vi "Path.vi"() -> (7 "path":T1)   [LabVIEW 2016]
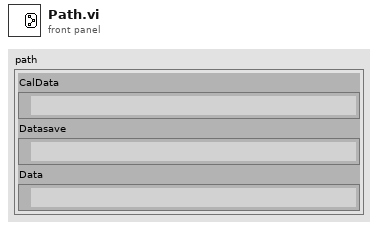
[diagram p1: front panel]
types:
  T1 = cluster{"CalData":path, "Datasave":path, "Data":path}
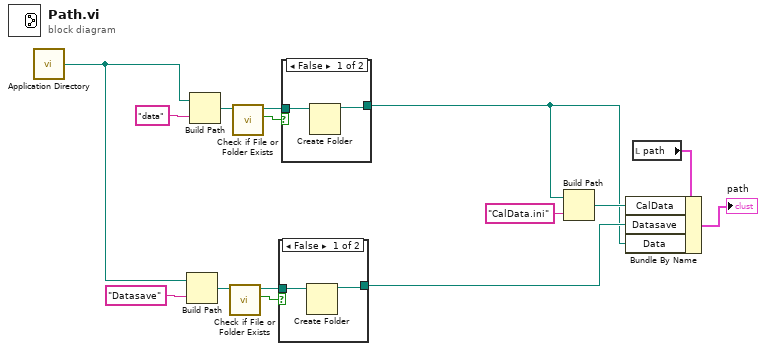
[diagram p0: block diagram]
diagram:
  n1 = call <vilib>:"Application Directory.vi"() -> ("Application Directory"=w3:path)
  n2 = Build Path(base path=w3, name or relative path="Datasave" ("名称或相对路径")) -> (appended path=w7:path)
  n3 = Build Path(base path=w3, name or relative path="data" ("名称或相对路径")) -> (appended path=w11:path)
  n4 = call <vilib>:"Check if File or Folder Exists.vi"("path"=w7) -> ("file or folder exists?"=w4:bool, "dup path"=w5:path)  [unwired: 8 in, 1 out]
  n5 = call <vilib>:"Check if File or Folder Exists.vi"("path"=w11) -> ("file or folder exists?"=w14:bool, "dup path"=w13:path)  [unwired: 8 in, 1 out]
  n6 = case shown="False" w4 {
    tunnel: [w16 w18] -> w2
    tunnel: w5 -> [w17 w18]
    frame False {
      n7 = Create Folder(path (use dialog)=w17) -> (created path=w16:path)  [unwired: 2 in, 2 out]
    }
    frame True {
    }
  }
  n8 = case shown="False" w14 {
    tunnel: [w19 w21] -> w1
    tunnel: w13 -> [w20 w21]
    frame False {
      n9 = Create Folder(path (use dialog)=w20) -> (created path=w19:path)  [unwired: 2 in, 2 out]
    }
    frame True {
    }
  }
  n10 = Build Path(base path=w1, name or relative path="CalData.ini" ("名称或相对路径")) -> (appended path=w9:path)
  n11 = local read "path"() -> (w15:T1)
  n12 = Bundle By Name(cluster=w15, "CalData"=w9, "Datasave"=w2, "Data"=w1) -> (→"path":T1)
